vi "MCLB_NameArray_Tests.vi"(11 "error in":errorcluster) -> (15 "error out":errorcluster)   [LabVIEW 2016, in "DronaTest.lvlib"]
uses:
  DronaTest.lvlib
  APIs/Stimulus/ControlValue/typedef/Name&Occurrence.ctl
  APIs/Stimulus/ControlValue/SetValueAuto.vi
  APIs/Stimulus/ControlValue/Controls/MC Listbox/SetValueByArrayName.vi
  APIs/Assert/AssertControlValue/Equal.vi
  APIs/Get/GetControlRef/GetControlRefByPath.vi
  <vilib>/addons/_JKI Toolkits/Caraya/classes/Test/Test.lvclass
  Drona.lvlib
  <vilib>/SLL Toolkit/SLL Debug/SLL Debug.lvlib
  APIs/Stimulus/ControlValue/ControlValue.lvlib
  APIs/Assert/AssertControlValue/AssertControlValue.lvlib
  <vilib>/addons/_JKI Toolkits/Caraya/classes/Assert/Assert.lvclass
  APIs/Stimulus/ControlValue/Controls/MC Listbox/StimulusMCListbox.lvlib
  APIs/Get/GetControlRef/GetControlRef.lvlib
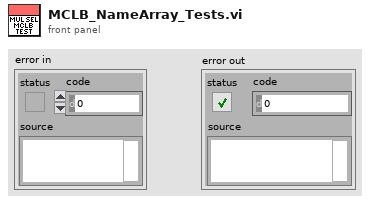
[diagram p1: front panel]
types:
  T1 = typedef "Drona.lvlib/ControlValue.lvlib/Name&Occurrence.ctl" = cluster{"ItemName":string, "Occurrence":i32}
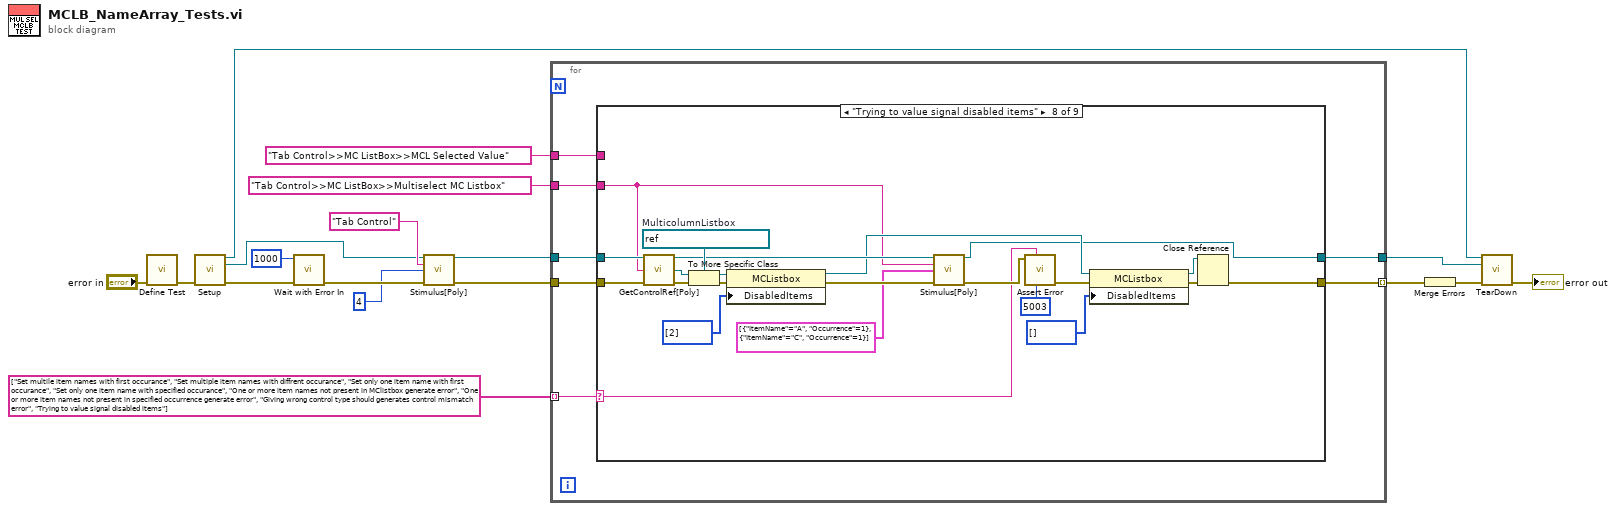
[diagram p0: block diagram]
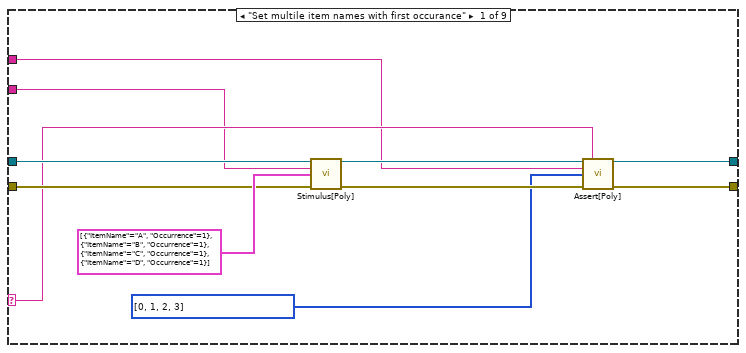
[diagram p2: hidden frame]
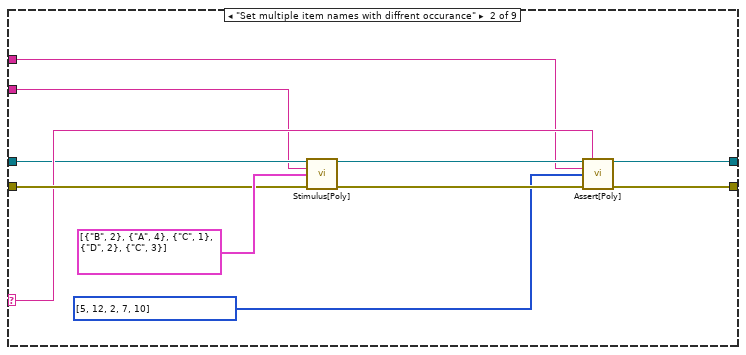
[diagram p3: hidden frame]
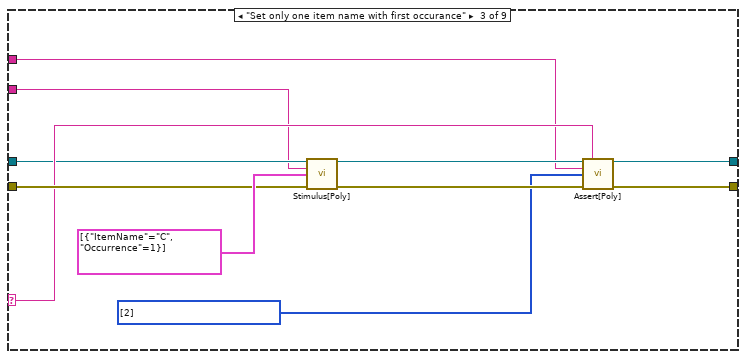
[diagram p4: hidden frame]
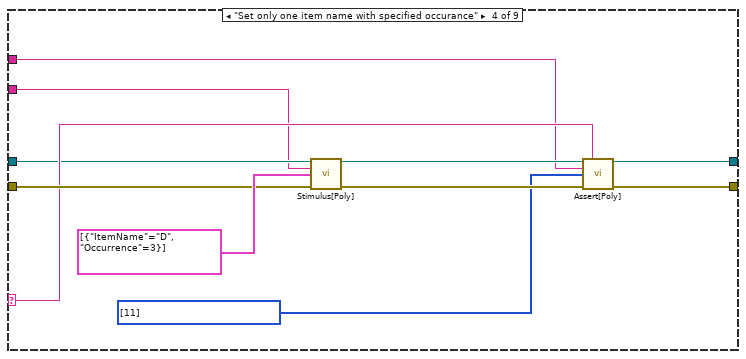
[diagram p5: hidden frame]
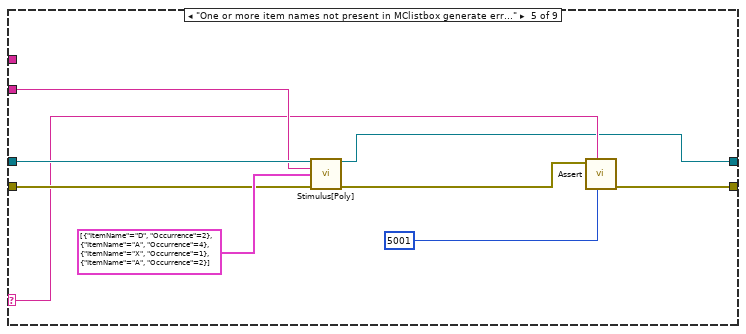
[diagram p6: hidden frame]
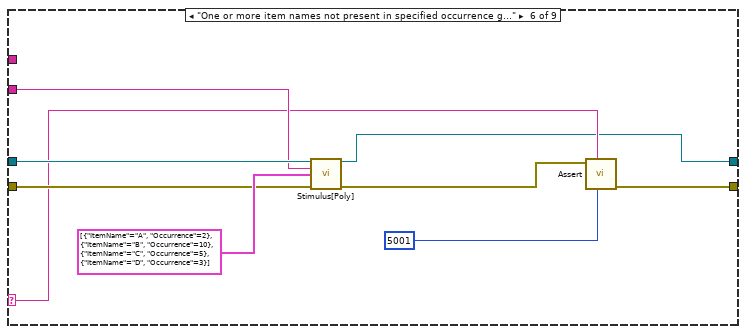
[diagram p7: hidden frame]
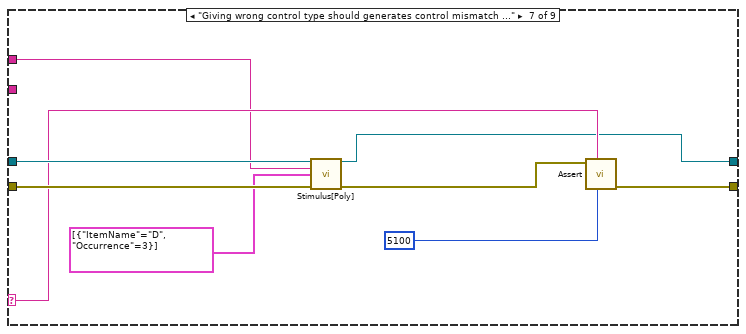
[diagram p8: hidden frame]
diagram:
  n1 = call <vilib>:"Define Test.vi"("error in (no error)"="error in") -> ("error out"=w7:errorcluster)  [unwired: 9 in, 1 out]
  n2 = call "Setup.vi"("error in (no error)"=w7) -> ("Application Ref"=w2:refnum<vi>, "VI out"=w6:refnum<vi>, "error out"=w5:errorcluster)  [unwired: 12 in]
  n3 = call <vilib>:"Wait with Error In.vi"("error in (no error)"=w5, "milliseconds to wait"=u32 1000) -> ("error out"=w16:errorcluster)  [unwired: 9 in]
  n4 = call-poly "Stimulus[Poly].vi"("VI Reference In"=w6, "Control Path"="Tab Control", "Value (Signaling)"=4, "error in"=w16) -> ("VI Reference Out"=w12:refnum<vi>, "error out"=w11:errorcluster)  [unwired: 10 in]
  n5 = for {
    tunnel: [w25] -> w10 mode=indexing
    tunnel: [w24] -> w3
    tunnel: string[] ["Set multile item names with first occurance", "Set multiple item names with diffrent occurance", "Set only one item name with first occurance", "Set only one item name with specified occurance", "One or more item names not present in MClistbox generate error", "One or more item names not present in specified occurrence generate error", "Giving wrong control type should generates control mismatch error", "Trying to value signal disabled items"] -> [w23] mode=indexing
    tunnel: w12 -> [w22]
    tunnel: w11 -> [w21]
    tunnel: "Tab Control>>MC ListBox>>Multiselect MC Listbox" ("Control Path") -> [w20]
    tunnel: "Tab Control>>MC ListBox>>MCL Selected Value" ("Control Path") -> [w19]
    n6 = case shown="\"Trying to value signal disabled items\"" w23 {
      selector: w23 -> [w28 w40 w51 w62 w71 w80 w91 w98 _]
      tunnel: [w36 w47 w58 w69 w73 w82 w93 w100 w119] -> w25
      tunnel: [w35 w46 w57 w68 w70 w79 w90 w99 w120] -> w24
      tunnel: w22 -> [w29 w39 w50 w61 w76 w85 w95 w102 w120]
      tunnel: w21 -> [w30 w41 w52 w63 w77 w86 w96 w103 w119]
      tunnel: w20 -> [w26 w38 w49 w60 w75 w84 _ w101 _]
      tunnel: w19 -> [w27 w37 w48 w59 _ _ w88 _ _]
      frame "Set multile item names with first occurance" {
        n7 = call-poly "Stimulus[Poly].vi"("VI Reference In"=w29, "Control Path"=w26, "Name Array"=T1[] [{"ItemName"="A", "Occurrence"=1}, {"ItemName"="B", "Occurrence"=1}, {"ItemName"="C", "Occurrence"=1}, {"ItemName"="D", "Occurrence"=1}], "Error In"=w30) -> ("VI Reference Out"=w33:refnum<vi>, "Error Out"=w34:errorcluster)  [unwired: 10 in]
        n8 = call-poly "Assert[Poly].vi"("VI Reference In"=w33, "Test Label"=w28, "Control Path"=w27, "Control Value"=i32[] [0, 1, 2, 3] ("Index Array"), "Error In"=w34) -> ("VI Reference Out"=w35:refnum<vi>, "Error Out"=w36:errorcluster)  [unwired: 8 in, 1 out]
      }
      frame "Set multiple item names with diffrent occurance" {
        n9 = call-poly "Stimulus[Poly].vi"("VI Reference In"=w39, "Control Path"=w38, "Name Array"=T1[] [{"ItemName"="B", "Occurrence"=2}, {"ItemName"="A", "Occurrence"=4}, {"ItemName"="C", "Occurrence"=1}, {"ItemName"="D", "Occurrence"=2}, {"ItemName"="C", "Occurrence"=3}], "Error In"=w41) -> ("VI Reference Out"=w44:refnum<vi>, "Error Out"=w45:errorcluster)  [unwired: 10 in]
        n10 = call-poly "Assert[Poly].vi"("VI Reference In"=w44, "Test Label"=w40, "Control Path"=w37, "Control Value"=i32[] [5, 12, 2, 7, 10] ("Index Array"), "Error In"=w45) -> ("VI Reference Out"=w46:refnum<vi>, "Error Out"=w47:errorcluster)  [unwired: 8 in, 1 out]
      }
      frame "Set only one item name with first occurance" {
        n11 = call-poly "Stimulus[Poly].vi"("VI Reference In"=w50, "Control Path"=w49, "Name Array"=T1[] [{"ItemName"="C", "Occurrence"=1}], "Error In"=w52) -> ("VI Reference Out"=w55:refnum<vi>, "Error Out"=w56:errorcluster)  [unwired: 10 in]
        n12 = call-poly "Assert[Poly].vi"("VI Reference In"=w55, "Test Label"=w51, "Control Path"=w48, "Control Value"=i32[] [2] ("Index Array"), "Error In"=w56) -> ("VI Reference Out"=w57:refnum<vi>, "Error Out"=w58:errorcluster)  [unwired: 8 in, 1 out]
      }
      frame "Set only one item name with specified occurance" {
        n13 = call-poly "Stimulus[Poly].vi"("VI Reference In"=w61, "Control Path"=w60, "Name Array"=T1[] [{"ItemName"="D", "Occurrence"=3}], "Error In"=w63) -> ("VI Reference Out"=w66:refnum<vi>, "Error Out"=w67:errorcluster)  [unwired: 10 in]
        n14 = call-poly "Assert[Poly].vi"("VI Reference In"=w66, "Test Label"=w62, "Control Path"=w59, "Control Value"=i32[] [11] ("Index Array"), "Error In"=w67) -> ("VI Reference Out"=w68:refnum<vi>, "Error Out"=w69:errorcluster)  [unwired: 8 in, 1 out]
      }
      frame "One or more item names not present in MClistbox generate error" {
        n15 = call-poly "Stimulus[Poly].vi"("VI Reference In"=w76, "Control Path"=w75, "Name Array"=T1[] [{"ItemName"="D", "Occurrence"=2}, {"ItemName"="A", "Occurrence"=4}, {"ItemName"="X", "Occurrence"=1}, {"ItemName"="A", "Occurrence"=2}], "Error In"=w77) -> ("VI Reference Out"=w70:refnum<vi>, "Error Out"=w74:errorcluster)  [unwired: 10 in]
        n16 = call-poly <vilib>:"Assert.vi"("error code (1)"=5001, "Label"=w71, "Error?"=w74) -> ("error out"=w73:errorcluster)  [unwired: 7 in, 1 out]
      }
      frame "One or more item names not present in specified occurrence generate error" {
        n17 = call-poly "Stimulus[Poly].vi"("VI Reference In"=w85, "Control Path"=w84, "Name Array"=T1[] [{"ItemName"="A", "Occurrence"=2}, {"ItemName"="B", "Occurrence"=10}, {"ItemName"="C", "Occurrence"=5}, {"ItemName"="D", "Occurrence"=3}], "Error In"=w86) -> ("VI Reference Out"=w79:refnum<vi>, "Error Out"=w83:errorcluster)  [unwired: 10 in]
        n18 = call-poly <vilib>:"Assert.vi"("error code (1)"=5001, "Label"=w80, "Error?"=w83) -> ("error out"=w82:errorcluster)  [unwired: 7 in, 1 out]
      }
      frame "Giving wrong control type should generates control mismatch error" {
        n19 = call-poly "Stimulus[Poly].vi"("VI Reference In"=w95, "Control Path"=w88, "Name Array"=T1[] [{"ItemName"="D", "Occurrence"=3}], "Error In"=w96) -> ("VI Reference Out"=w90:refnum<vi>, "Error Out"=w94:errorcluster)  [unwired: 10 in]
        n20 = call-poly <vilib>:"Assert.vi"("error code (1)"=5100, "Label"=w91, "Error?"=w94) -> ("error out"=w93:errorcluster)  [unwired: 7 in, 1 out]
      }
      frame "Trying to value signal disabled items" {
        w115 = refnum<vi> refnum  # MulticolumnListbox
        n21 = call-poly "GetControlRef[Poly].vi"("VI Reference In"=w102, "Control Path"=w101, "error In"=w103) -> ("VI Reference Out"=w111:refnum<vi>, "Ctl Refnum"=w116:refnum<vi>, "error out"=w118:errorcluster)  [unwired: 10 in]
        n22 = To More Specific Class(target class=w115, reference=w116, error in=w118) -> (specific class reference=w114:refnum<vi>, error out=w117:errorcluster)
        n23 = property class="MCListbox"(reference=w114, error in=w117, "DisabledItems"=i32[] [2] ("Disabled Items")) -> (reference out=w109:refnum<vi>, error out=w112:errorcluster)
        n24 = call-poly "Stimulus[Poly].vi"("VI Reference In"=w111, "Control Path"=w101, "Name Array"=T1[] [{"ItemName"="A", "Occurrence"=1}, {"ItemName"="C", "Occurrence"=1}], "Error In"=w112) -> ("VI Reference Out"=w99:refnum<vi>, "Error Out"=w106:errorcluster)  [unwired: 10 in]
        n25 = call <vilib>:"Assert Error.vi"("error code (1)"=5003, "Label"=w98, "Error?"=w106) -> ("error out"=w105:errorcluster)  [unwired: 7 in, 1 out]
        n26 = property class="MCListbox"(reference=w109, error in=w105, "DisabledItems"=i32[] [] ("Disabled Items")) -> (reference out=w107:refnum<vi>, error out=w110:errorcluster)
        n27 = Close Reference(reference=w107, error in (no error)=w110) -> (error out=w100:errorcluster)
      }
      frame Default {
      }
    }
  }
  n28 = Merge Errors(w10) -> (w4:errorcluster)
  n29 = call "TearDown.vi"("Application Ref"=w2, "VI in"=w3, "error in (no error)"=w4) -> ("error out"=→"error out":errorcluster)  [unwired: 12 in]
